vi "get_XYZ.vi"(0 "Actuator cluster in":T1={"Actuator COM"="COM14", "Actuator type"=enum."Scientifica"}, 11 "error in":errorcluster) -> (4 "Actuator cluster out":T1={"Actuator COM"="COM14", "Actuator type"=enum."Scientifica"}, 6 "X pos (steps)":i32, 8 "Y pos (steps)":i32, 10 "Z pos (steps)":i32, 15 "error out":errorcluster)   [LabVIEW 2019]
uses:
  controls/actuator_cluster.ctl
  controls/actuator_type.ctl
panel:
  # "ACTUATOR GET XYZ (STEPS)"
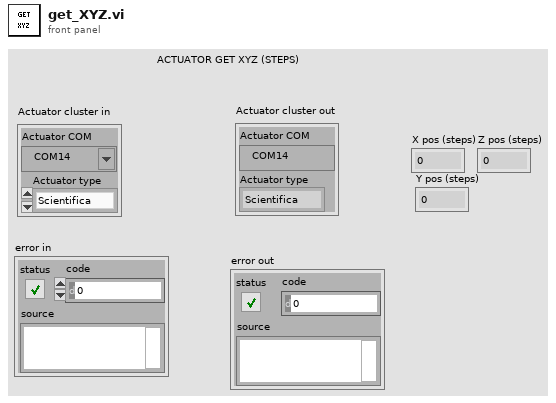
[diagram p1: front panel]
types:
  T1 = typedef "actuator_cluster.ctl" = cluster{"Actuator COM":refnum<visa-resource-name>, "Actuator type":T2}
  T2 = typedef "actuator_type.ctl" = enum16{"Scientifica", "Sutter", "Demo", "Off"}
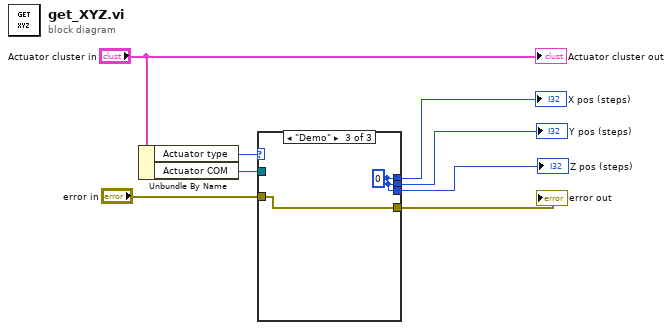
[diagram p0: block diagram]
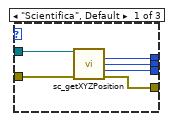
[diagram p2: hidden frame]
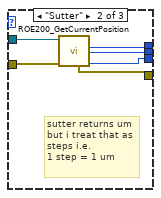
[diagram p3: hidden frame]
diagram:
  n1 = Unbundle By Name("Actuator cluster in") -> ("Actuator type"=w8:T2, "Actuator COM"=w7:refnum<visa-resource-name>)
  n2 = case shown="\"Demo\"" w8 {
    tunnel: w7 -> [w14 w20 _]
    tunnel: "error in" -> [w13 w19 w21]
    tunnel: [w12 w16 w21] -> w5
    tunnel: [w11 w18 w22] -> w4
    tunnel: [w10 w17 w22] -> w3
    tunnel: [w9 w15 w22] -> w2
    frame "Scientifica", Default {
      n3 = call "sc_getXYZPosition.vi"("VISA handle 2"=w14, "error in (no error) 2"=w13) -> ("X pos (steps)"=w11:i32, "Y pos (steps)"=w10:i32, "Z pos (steps)"=w9:i32, "error out 2"=w12:errorcluster)  [unwired: 9 in, 1 out]
    }
    frame "Sutter" {
      # "sutter returns um\nbut i treat that as\nsteps i.e. \n1 step = 1 um"
      n4 = call "ROE200_GetCurrentPosition.vi"("error in (no error)"=w19, "VISA resource name"=w20) -> ("Z Position"=w15:u32, "Y Position"=w17:u32, "X Position"=w18:u32, "error out"=w16:errorcluster)  [unwired: 3 in, 3 out]
    }
    frame "Demo" {
      w22 = u32 0 ("X Position")
    }
  }
  "error out" <- w5
  "X pos (steps)" <- w4
  "Y pos (steps)" <- w3
  "Z pos (steps)" <- w2
  "Actuator cluster out" <- "Actuator cluster in"
